vi "CMD_execute.vi"(2 "Inst_info":T1, 3 "WorkFilePath":path, 4 "Indexes":u64[](array[numeric])) -> ()   [LabVIEW 2013]
uses:
  <vilib>/addons/h5labview2/base/lib_path.vi
  <vilib>/addons/h5labview2/base/H5Equery.vi
  <vilib>/addons/h5labview2/dataset/H5Dread.llb/H5Dread.xnode
  <vilib>/addons/h5labview2/base/hid_t.ctl
  <vilib>/addons/h5labview2/dataset/H5D.lvlib
  <vilib>/addons/h5labview2/space/H5S.lvlib
  <vilib>/addons/h5labview2/file/H5F.lvlib
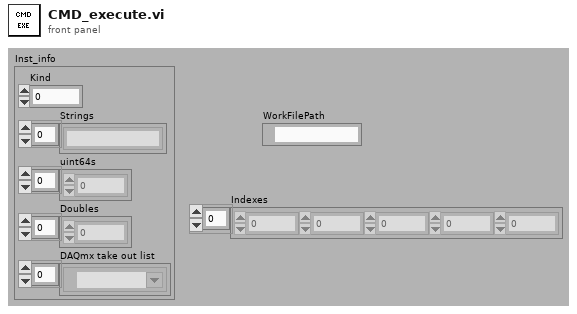
[diagram p1: front panel]
types:
  T1 = cluster{"Kind":u16, "Strings":string[], "uint64s":u64[], "Doubles":dbl[], "DAQmx take out list":refnum<k21>[]}
  T2 = typedef "hid_t.ctl" = i32
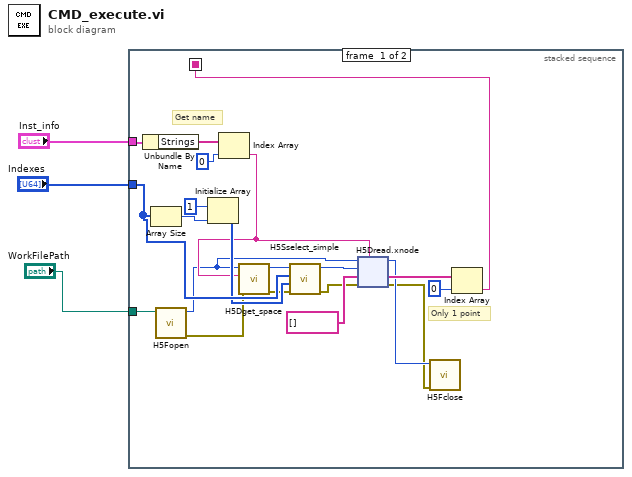
[diagram p0: block diagram]
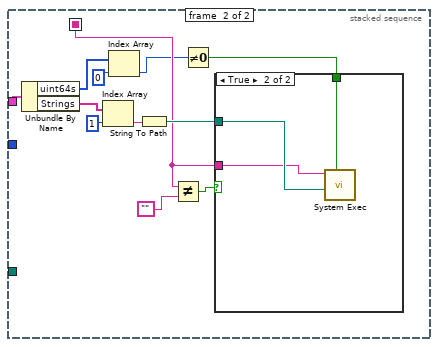
[diagram p2: hidden frame]
diagram:
  n1 = stacked-sequence {
    seq-local: [w12 _] -> [_ w44]
    tunnel: "Inst_info" -> [w24 w51]
    tunnel: "Indexes" -> [w14 _]
    tunnel: "WorkFilePath" -> [w10 _]
    frame #0 {
      # "Only 1 point"
      # "Get name"
      n2 = Unbundle By Name(w24) -> ("Strings"=w23:string[])
      n3 = Array Size(array=w14) -> (size(s)=w16:i32)
      n4 = call <vilib>:"H5Fopen.vi"("path"=w10) -> ("error out"=w9:errorcluster, "ref out"=w8:T2)  [unwired: 9 in]
      n5 = Initialize Array(u32 1, w16) -> (w13:u32[])
      n6 = Index Array(array=w23, index=0) -> (element=w11:string)
      n7 = call <vilib>:"H5Dget_space.vi"("error in (no error)"=w9, "obj (.)"=w11, "ref in"=w8) -> ("error out"=w7:errorcluster, "space out"=w21:T2)  [unwired: 7 in]
      n8 = call <vilib>:"H5Sselect_simple.vi"("error in (no error)"=w7, "count"=w13, "start"=w14, "space in"=w21) -> ("error out"=w6:errorcluster, "space out"=w20:T2)  [unwired: 6 in]
      n9 = xnode "H5Dread.xnode"("dataset name (this)"=w11, "error in (no error)"=w6, "default"=string[] [], "file space"=w20, "ref in"=w8) -> ("error out"=w4:errorcluster, "data"=w18:string[], "ref out"=w5:T2)  [unwired: 1 in, 1 out]
      n10 = call <vilib>:"H5Fclose.vi"("error in (no error)"=w4, "ref"=w5) -> ()  [unwired: 9 in, 1 out]
      n11 = Index Array(array=w18, index=0) -> (element=w12:string)
    }
    frame #1 {
      n12 = Unbundle By Name(w51) -> ("uint64s"=w43:u64[], "Strings"=w50:string[])
      n13 = Index Array(array=w50, index=1) -> (element=w48:string)
      n14 = Index Array(array=w43, index=0) -> (element=w41:u64)
      n15 = String To Path(string=w48) -> (path=w45:path)
      n16 = Not Equal?(x=w44, y="") -> (x != y?=w47:bool)
      n17 = Not Equal To 0?(x=w41) -> (x != 0?=w40:bool)
      n18 = case shown="True" w47 {
        tunnel: w45 -> [_ w54]
        tunnel: w44 -> [_ w53]
        tunnel: w40 -> [_ w52]
        frame False {
        }
        frame True {
          n19 = call <vilib>:"System Exec.vi"("wait until completion? (T)"=w52, "working directory"=w54, "command line"=w53) -> ()  [unwired: 5 in, 4 out]
        }
      }
    }
  }
